vi "Set Stage Acceleration.vi"(8 "error in":errorcluster, 10 "Acceleration":dbl, 11 ".NET Refnum in":refnum<k24>) -> (0 "error out":errorcluster, 3 ".NET Refnum out":refnum<k24>)   [LabVIEW 2013, in "ThorlabsLTS.lvclass"]
uses:
  ThorlabsLTS.lvclass
  C:/GEECS/Developers Version/source/Device Driver/ThorLabsLTS/Thorlabs.MotionControl.IntegratedStepperMotorsCLI.dll
  Thorlabs.MotionControl.IntegratedStepperMotorsCLI.dll
  C:/GEECS/Developers Version/source/Device Driver/ThorLabsLTS/Thorlabs.MotionControl.GenericMotorCLI.dll
  Thorlabs.MotionControl.GenericMotorCLI.dll
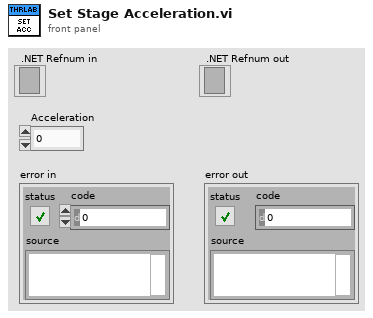
[diagram p1: front panel]
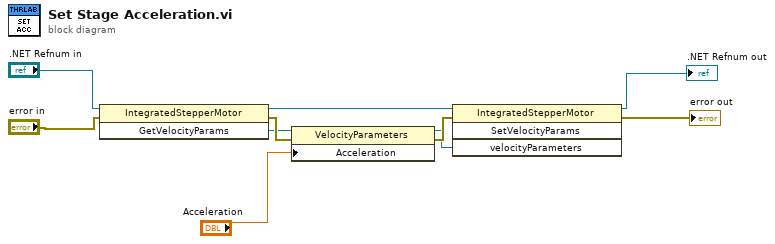
[diagram p0: block diagram]
diagram:
  n1 = invoke class="IntegratedStepperMotor" method="GetVelocityParams"(reference=".NET Refnum in", error in="error in") -> (reference out=w6:refnum<k24>, error out=w3:errorcluster, "GetVelocityParams"=w2:refnum<k24>)  [unwired: 1 in]
  n2 = property class="VelocityParameters"(reference=w2, error in=w3, "Acceleration"="Acceleration") -> (reference out=w4:refnum<k24>, error out=w5:errorcluster)
  n3 = invoke class="IntegratedStepperMotor" method="SetVelocityParams"(reference=w6, error in=w5, "velocityParameters"=w4) -> (reference out=→".NET Refnum out":refnum<k24>, error out=→"error out":errorcluster)  [unwired: 1 in, 2 out]
